vi "Set ICP2-DO Changed bit.vi"(7 "Wait (F)":bool, 8 "error in (no error)":errorcluster, 9 "Value":bool, 10 "DO Channel":T1, 11 "IO in":refnum<class "IO.lvclass">) -> (0 "error out":errorcluster, 3 "IO out":refnum<class "IO.lvclass">)   [LabVIEW 2022 SP3, in "IO.lvclass"]
uses:
  IO.lvclass
  Typedefs/ICP2-DO Channel Names.ctl
  Typedefs/API Command Cluster.ctl
  Typedefs/API Command Enum.ctl
  Typedefs/DO Value API Data.ctl
  Typedefs/Device Names.ctl
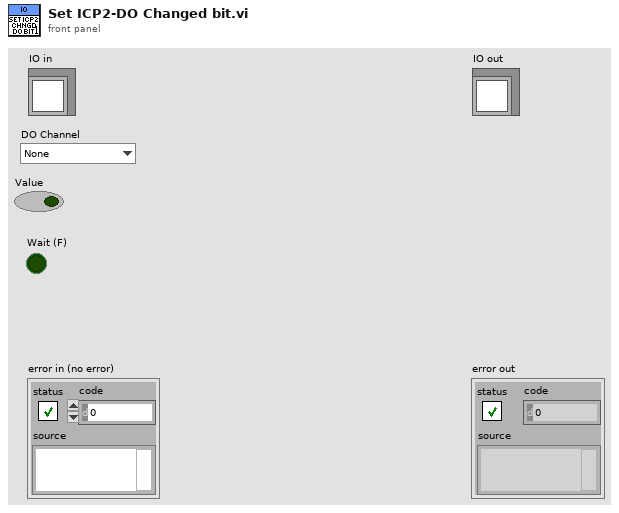
[diagram p1: front panel]
types:
  T1 = typedef "IO.lvclass/ICP2-DO Channel Names.ctl" = enum16{"None", "Meniscus Valve Open - R1", "Meniscus Valve Open - R2", "Meniscus Valve Open - R3", "Meniscus Valve Open - R4", "Meniscus Valve Open - R5", "Meniscus Valve Open - R6", "Ink Flow Valve Open - R1", "Ink Flow Valve Open - R2", "Ink Flow Valve Open - R3", "Ink Flow Valve Open - R4", "Ink Flow Valve Open - R5", "Ink Flow Valve Open - R6", "SW_LED - Ink Valve - R1", "SW_LED - Ink Valve - R2", "SW_LED - Ink Valve - R3", "Recirc Pump On - R1", "Recirc Pump On - R2", "Recirc Pump On - R3", "Recirc Pump On - R4", "Recirc Pump On - R5", "Recirc Pump On - R6", "SW_LED - Ink Valve - R4", "SW_LED - Ink Valve - R5", "SW_LED - Ink Valve - R6"}
  T2 = typedef "IO.lvclass/Device Names.ctl" = enum16{"ICP1-DO", "ICP2-DI", "ICP2-DO", "ICP1-AI", "ICP1-AO", "ICP2-AO"}
  T3 = typedef "IO.lvclass/DO Value API Data.ctl" = cluster{"Device Name":T2, "Value":bool, "Index":i32}
  T4 = typedef "IO.lvclass/API Command Enum.ctl" = enum16{"Set DO Value", "Set AO Value", "Purge PH"}
  T5 = typedef "IO.lvclass/API Command Cluster.ctl" = cluster{"Command":T4, "Arguments":string, "Data":variant}
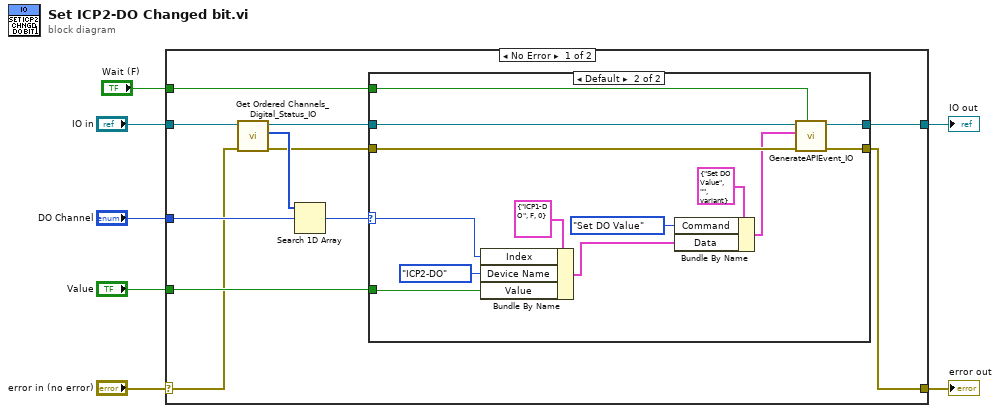
[diagram p0: block diagram]
diagram:
  n1 = case shown="No Error" "error in (no error)" {
    selector: "error in (no error)" -> [w11 w35]
    tunnel: [w10 w35] -> w6
    tunnel: [w14 w34] -> w4
    tunnel: "IO in" -> [w18 w34]
    tunnel: "DO Channel" -> [w16 _]
    tunnel: "Value" -> [w13 _]
    tunnel: "Wait (F)" -> [w8 _]
    frame No Error {
      n2 = call-dynamic "Get Ordered Channels_Digital_Status_IO.vi"("error in (no error)"=w11, "IO in"=w18) -> ("error out"=w12:errorcluster, "Ordered ICP2-DO Channels"=w17:T1[], "IO out"=w15:refnum<class "IO.lvclass">)  [unwired: 5 in, 2 out]
      n3 = Search 1D Array(1D array=w17, element=w16) -> (index of element=w9:i32)  [unwired: 1 in]
      n4 = case shown="Default" w9 {
        selector: w9 -> [_ w25]
        tunnel: w15 -> [w20 w21]
        tunnel: [w20 w32] -> w14
        tunnel: w13 -> [_ w26]
        tunnel: w12 -> [w19 w33]
        tunnel: [w19 w31] -> w10
        tunnel: w8 -> [_ w22]
        frame -1 {
        }
        frame Default {
          n5 = Bundle By Name(cluster=T3 {"Device Name"=enum."ICP1-DO", "Value"=FALSE, "Index"=0} ("DO Value Input"), "Index"=w25, "Device Name"=Device_Names."ICP2-DO", "Value"=w26) -> (w24:T3)
          n6 = Bundle By Name(cluster=T5 {"Command"=enum."Set DO Value", "Arguments"="", "Data"=variant} ("API Command Cluster"), "Command"=API_Command_Enum."Set DO Value", "Data"=w24) -> (w28:T5)
          n7 = call "GenerateAPIEvent_IO.vi"("Wait (F)"=w22, "error in (no error)"=w33, "API Command Cluster"=w28, "IO.lvclass"=w21) -> ("error out"=w31:errorcluster, "IO.lvclass out"=w32:refnum<class "IO.lvclass">)  [unwired: 6 in]
        }
      }
    }
    frame Error {
    }
  }
  "error out" <- w6
  "IO out" <- w4
